vi "Test Simulation File.vi"() -> ()   [LabVIEW 2012]
uses:
  Type/_File Command.ctl
panel:
  out "SpecSize":i32
  out "MassSize":i32
  out "sum":u32
  out "Spectrum":u32[](array[numeric])
  out "Mass":dbl[](array[numeric])
  out "TIC":u32
  in  "RetTime(mS)":i64=1
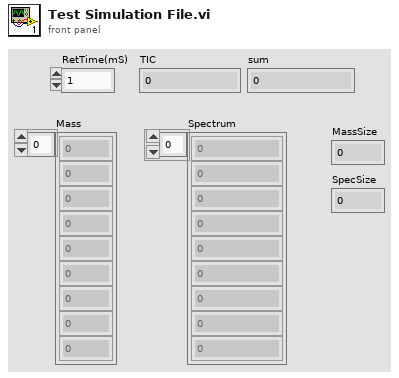
[diagram p1: front panel]
types:
  T1 = typedef "_File Command.ctl" = enum16{"No Command", "Open", "Open Read", "Write", "Get Spectrum", "Close"}
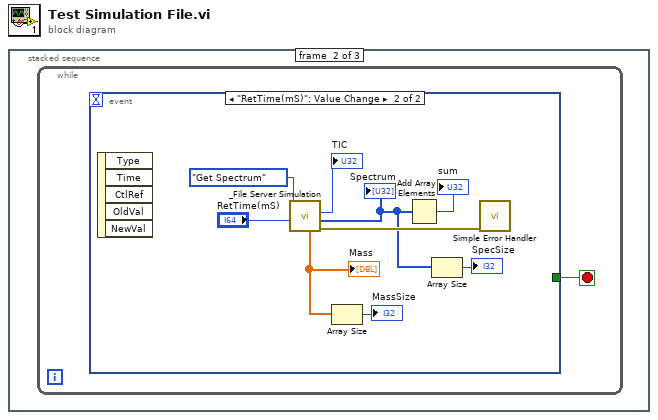
[diagram p0: block diagram]
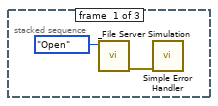
[diagram p2: hidden frame]
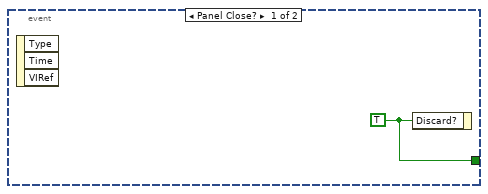
[diagram p3: hidden frame]
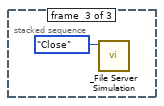
[diagram p4: hidden frame]
diagram:
  n1 = stacked-sequence {
    frame #0 {
      n2 = call "_File Server Simulation.vi"("FileCommand"=_File_Command."Open") -> ("ErrorOut"=w1:errorcluster)  [unwired: 7 in, 3 out]
      n3 = call <vilib>:"Simple Error Handler.vi"("error in (no error)"=w1) -> ()  [unwired: 4 in, 5 out]
    }
    frame #1 {
      n4 = while {
        stop <- w3 stop-if-true
        n5 = event shown="[1] \"RetTime(mS)\": Value Change" {
          selector: _ -> [_ _]
          dyn-events: _ -> [_ _]
          timeout: _ -> [_ _]
          tunnel: [w4 _] -> w3
          event Panel Close? {
            w4 = TRUE ("Discard?")
            n6 = event-data() -> ()  [unwired: 1 in, 3 out]
            n7 = event-data("Discard?"=w4) -> ()  [unwired: 1 in, 1 out]
          }
          event "RetTime(mS)": Value Change {
            n8 = event-data() -> ()  [unwired: 1 in, 5 out]
            n9 = call "_File Server Simulation.vi"("RetTime(mS)"="RetTime(mS)", "FileCommand"=_File_Command."Get Spectrum") -> ("ErrorOut"=w11:errorcluster, "Spectrum"=w5:u32[], "TIC"=→"TIC":u32, "Mass"=w8:dbl[])  [unwired: 6 in]
            "Mass" <- w8
            "Spectrum" <- w5
            n10 = Array Size(array=w8) -> (size(s)=→"MassSize":i32)
            n11 = Add Array Elements(numeric array=w5) -> (sum=→"sum":u32)
            n12 = Array Size(array=w5) -> (size(s)=→"SpecSize":i32)
            n13 = call <vilib>:"Simple Error Handler.vi"("error in (no error)"=w11) -> ()  [unwired: 4 in, 5 out]
          }
        }
      }
    }
    frame #2 {
      n14 = call "_File Server Simulation.vi"("FileCommand"=_File_Command."Close") -> ()  [unwired: 7 in, 4 out]
    }
  }
